vi "Physical Channels to Number of channels.vi"(8 "error in (no error)":errorcluster, 11 "Physical Channel in":refnum<k21>) -> (0 "error out":errorcluster, 2 "Array of Strings":string[](array[string]), 3 "Number of Channels":i32)   [LabVIEW 2016]
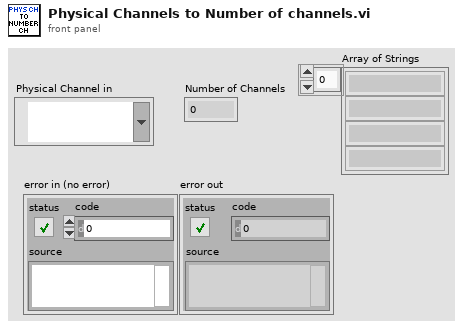
[diagram p1: front panel]
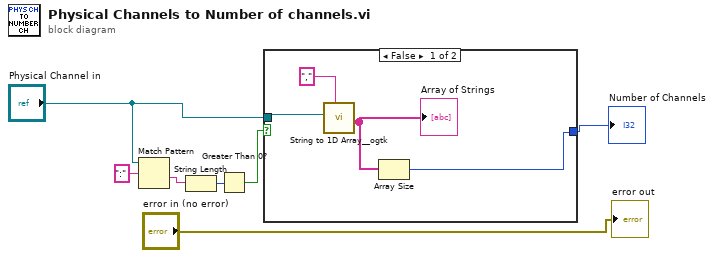
[diagram p0: block diagram]
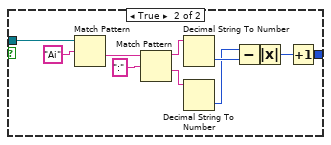
[diagram p2: hidden frame]
diagram:
  n1 = Match Pattern(string="Physical Channel in", regular expression=":") -> (after substring=w4:string)  [unwired: 1 in, 3 out]
  n2 = String Length(string=w4) -> (length=w3:i32)
  n3 = Greater Than 0?(x=w3) -> (x > 0?=w2:bool)
  n4 = case shown="False" w2 {
    tunnel: [w8 w22] -> w7
    tunnel: "Physical Channel in" -> [w11 w12]
    frame False {
      n5 = call "String to 1D Array__ogtk.vi"("delimiter (Tab)"=",", "string"=w11) -> ("Array of Strings"=w9:string[])  [unwired: 9 in]
      "Array of Strings" <- w9
      n6 = Array Size(array=w9) -> (size(s)=w8:i32)
    }
    frame True {
      n7 = Match Pattern(string=w12, regular expression="Ai") -> (after substring=w15:string)  [unwired: 1 in, 3 out]
      n8 = Match Pattern(string=w15, regular expression=":") -> (before substring=w17:string, after substring=w18:string)  [unwired: 1 in, 2 out]
      n9 = Decimal String To Number(string=w17) -> (number=w20:i32)  [unwired: 2 in, 1 out]
      n10 = Decimal String To Number(string=w18) -> (number=w19:i32)  [unwired: 2 in, 1 out]
      n11 = Subtract(x=w19, y=w20) -> (x-y=w21:i32)
      n12 = Absolute Value(x=w21) -> (abs(x)=w13:i32)
      n13 = Increment(x=w13) -> (x+1=w22:i32)
    }
  }
  "Number of Channels" <- w7
  "error out" <- "error in (no error)"
